vi "Main.vi"() -> ()   [LabVIEW 2015]
doc: "This template is for the Queued Message Handler design pattern.\n\nThe Event Handling Loop generates messages based on user interface actions.\n\nThe Message Handling Loop processes messages generated by the Event Handling Loop, or by other messages. The messages are string values, so new messages can be added easily to the Message Cases case structure in the Message Handling Loop. Each message cluster can also provide an optional value for Message Data, which is a variant that can be converted to whatever message-specific data is required."
uses:
  support/Type Definitions/UI Data.ctl
  support/Message Queue/Message Queue.lvlib
  Support/User Event - EHL Stop/User Event - EHL Stop.lvlib
  support/Message Queue/Enqueue Message (Single).vi
  <vilib>/ErrorRing/Error Ring.xnode
  Model/Model.lvlib
  PLC/PLC.lvlib
  support/Status Logger/Status Log.ctl
  support/Global names.vi
  <vilib>/Utility/error.llb/Error Cluster From Error Code.vi
panel:
  out "Power status":bool
  in  "Abort":bool
  in  "Stop Line":bool
  in  "Start Line":bool
  out "Status":string
  in  "Tab Control":enum32{"Simulation"}(tab)
  in  "Power switch":bool
  in  "Positon":dbl(slide) scale=0.0..20.0
  in  "Dispose":bool
  in  "Pump":bool
  in  "Flow [l/s]":dbl=10.0
  in  "Exit":bool
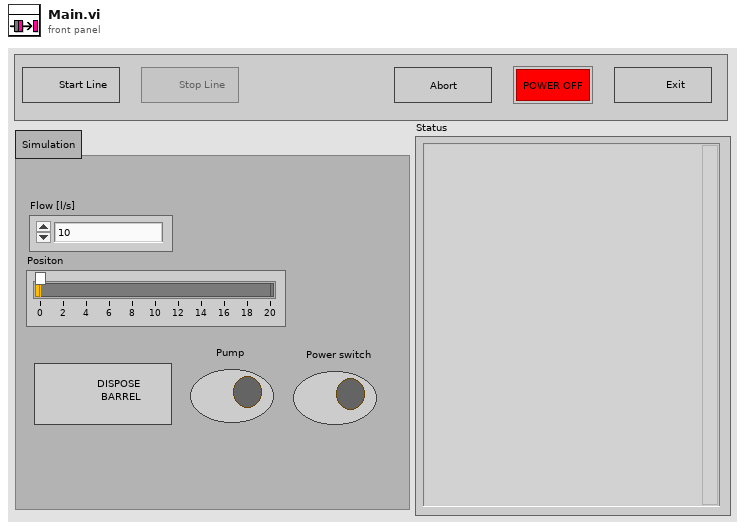
[diagram p1: front panel]
types:
  T1 = typedef "Status Log.ctl" = enum16{"Close file", "Open Status file", "Add Status", "Show Status File"}
  T2 = typedef "UI Data.ctl" = cluster{"Start Line Ref":refnum<vi>, "Stop Line Ref":refnum<vi>, "Data Display Ref":refnum<vi>, "Exit Button Ref":refnum<vi>, "Pump Ref":refnum<vi>, "Dispose Ref":refnum<vi>, "Flow Ref":refnum<vi>, "Position Ref":refnum<vi>, "Tab Ref":refnum<vi>, "Abort":refnum<vi>, "Power status":refnum<vi>, "Power switch":refnum<vi>}
  T3 = typedef "Notifiers.lvlib/Notifiers.ctl" = cluster{"PLC":refnum<notifier>, "Model":refnum<notifier>}
  T4 = typedef "Message Queue.lvlib/All Message Queues.ctl" = cluster{"UI":refnum<queue>, "Model":refnum<queue>, "PLC":refnum<queue>}
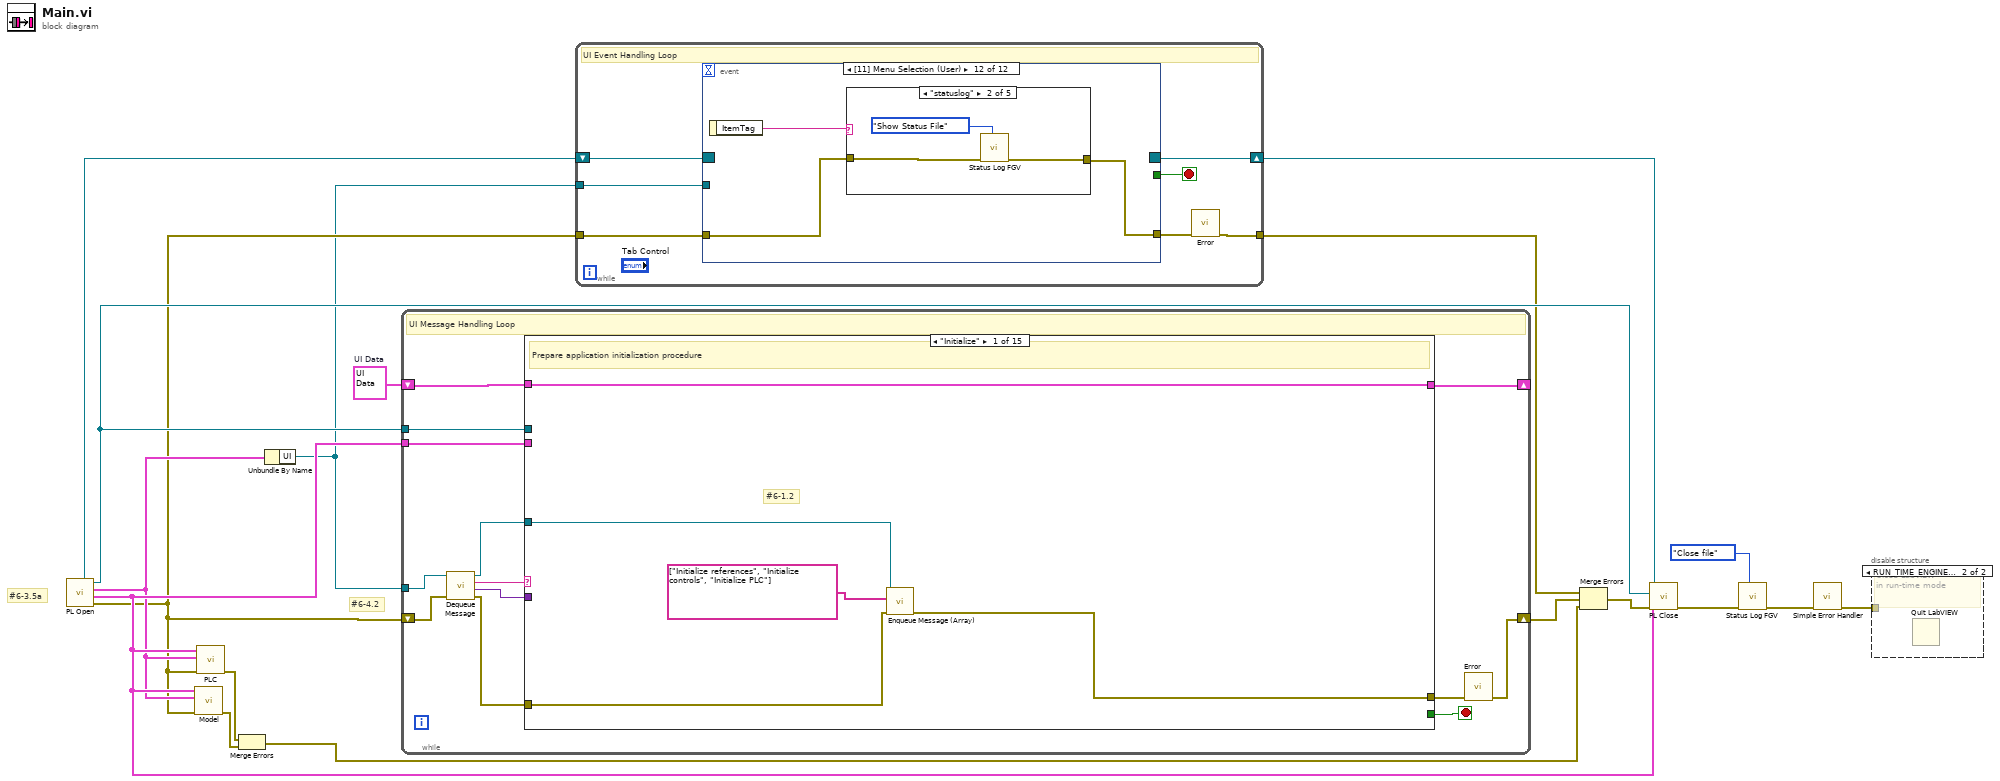
[diagram p0: block diagram]
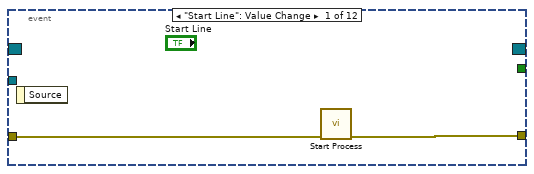
[diagram p2: hidden frame]
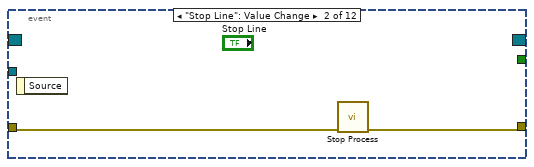
[diagram p3: hidden frame]
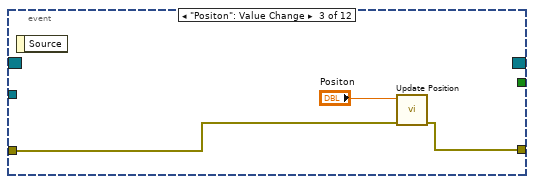
[diagram p4: hidden frame]
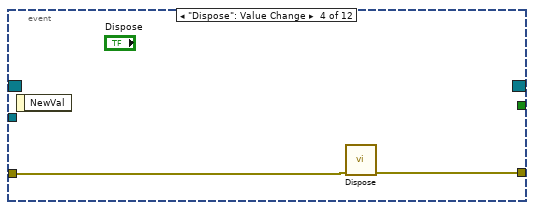
[diagram p5: hidden frame]
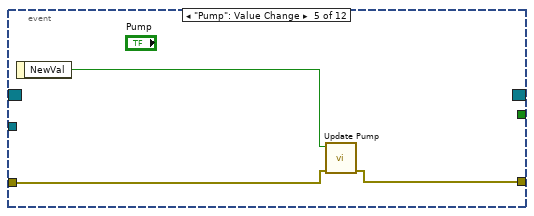
[diagram p6: hidden frame]
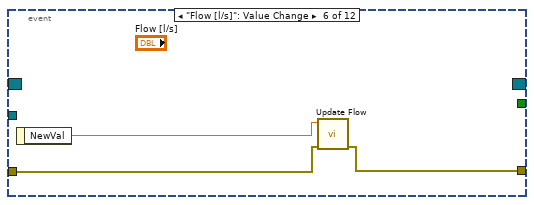
[diagram p7: hidden frame]
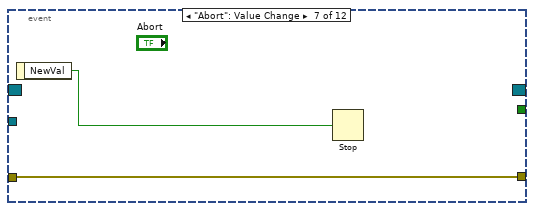
[diagram p8: hidden frame]
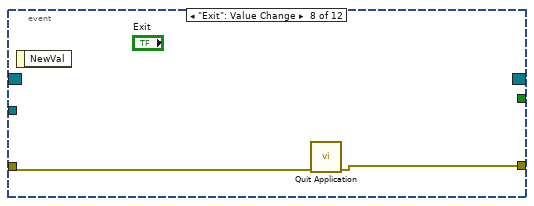
[diagram p9: hidden frame]
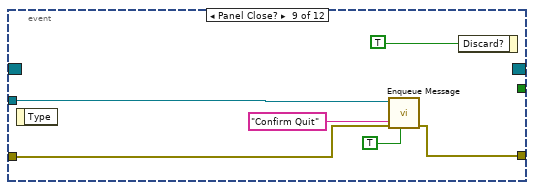
[diagram p10: hidden frame]
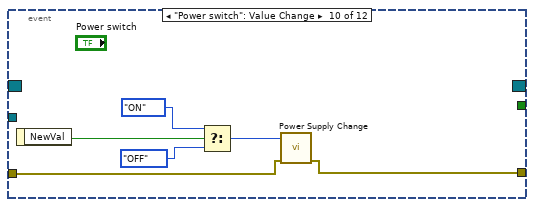
[diagram p11: hidden frame]
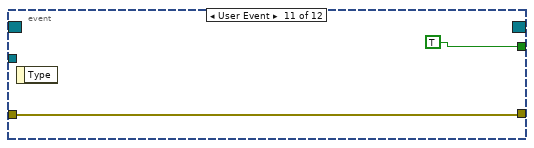
[diagram p12: hidden frame]
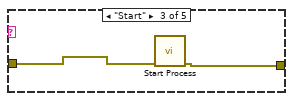
[diagram p14: hidden frame]
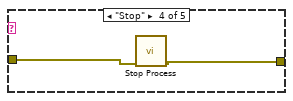
[diagram p15: hidden frame]
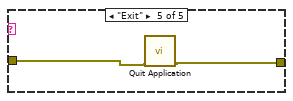
[diagram p16: hidden frame]
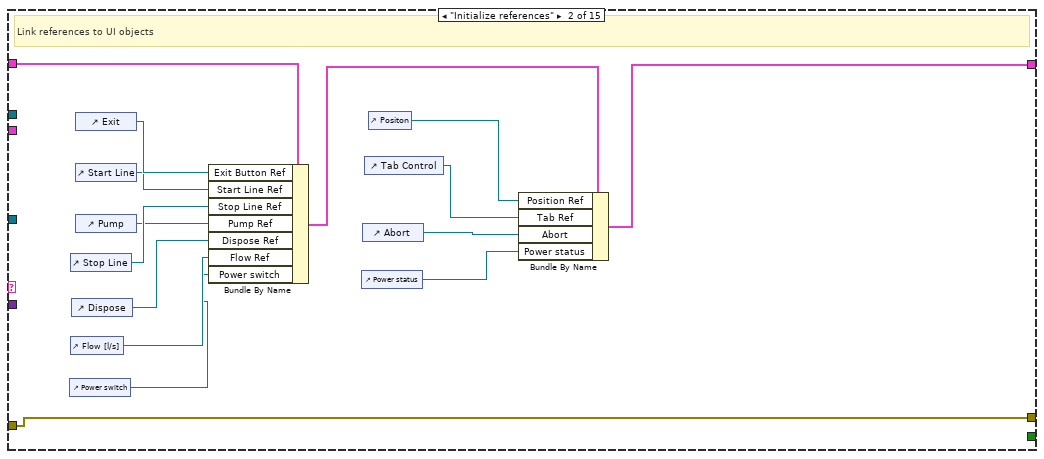
[diagram p18: hidden frame]
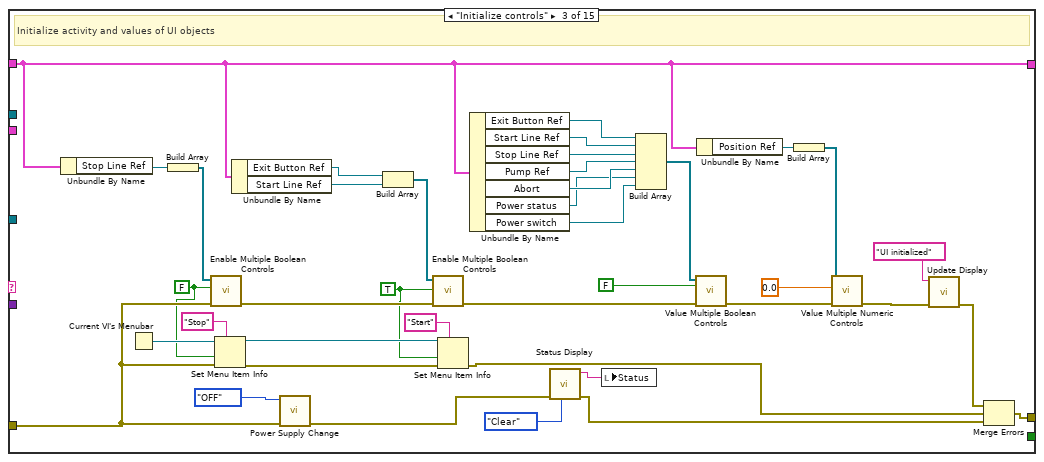
[diagram p19: hidden frame]
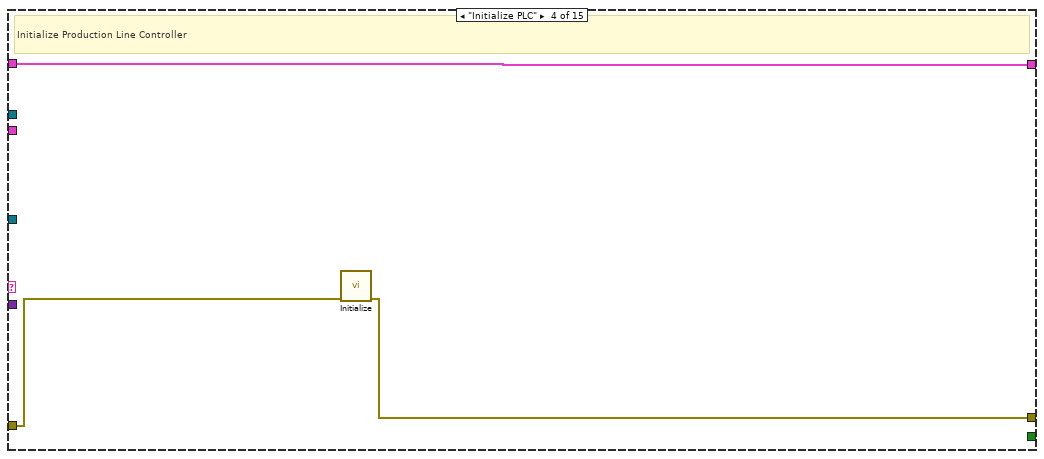
[diagram p20: hidden frame]
diagram:
  w17 = T2 {"Start Line Ref"=refnum, "Stop Line Ref"=refnum, "Data Display Ref"=refnum, "Exit Button Ref"=refnum, "Pump Ref"=refnum, "Dispose Ref"=refnum, "Flow Ref"=refnum, "Position Ref"=refnum, "Tab Ref"=refnum, "Abort"=refnum, "Power status"=refnum, "Power switch"=refnum}  # UI Data
  # "#6-3.5a"
  # "#6-4.2"
  n1 = call "PL Open.vi"() -> ("error out"=w2:errorcluster, "Notifiers"=w7:T3, "Queues"=w6:T4, "User Event"=w15:refnum<user-event>, "Event Registration Refnum"=w9:refnum<event-registration>)  [unwired: 7 in]
  n2 = call "Model.vi"("error in"=w2, "Queues"=w6, "Notifiers"=w7) -> ("error out"=w4:errorcluster)  [unwired: 8 in]
  n3 = call "PLC.vi"("error in"=w2, "Message Queues"=w6, "Notifiers"=w7) -> ("error out"=w5:errorcluster)  [unwired: 8 in]
  n4 = Merge Errors(w5, w4) -> (w3:errorcluster)
  n5 = Unbundle By Name(w6) -> ("UI"=w1:refnum<queue>)
  n6 = while {
    shift-right: [w30] -> _
    shift-left: w17 -> [w31]
    tunnel: w15 -> [w28]
    tunnel: w7 -> [w24]
    shift-right: [w20] -> w13
    shift-left: w2 -> [w27]
    tunnel: w1 -> [w22]
    stop <- w29 stop-if-true
    # "UI Message Handling Loop"
    n7 = call "Dequeue Message.vi"("error in (no error)"=w27, "Message Queue"=w22) -> ("error out"=w26:errorcluster, "Message Data"=w23:variant, "Message"=w19:string, "dup Message Queue"=w25:refnum<queue>)  [unwired: 6 in]
    n8 = case "Message Cases" shown="\"Initialize\"" w19 {
      selector: w19 -> [_ _ _ _ _ _ _ _ _ _ _ _ _ _ w245]
      tunnel: w25 -> [w34 _ _ _ _ _ _ _ _ _ w191 w197 w233 _ _]
      tunnel: w26 -> [w35 w40 w60 w91 w107 w125 w138 w153 w181 w183 w192 w199 w216 w240 _]
      tunnel: [w33 w40 w69 w92 w106 w127 w140 w154 w175 w182 w189 w196 w220 w234 w244] -> w21
      tunnel: w31 -> [w36 w51 w77 w93 w112 w137 w145 w157 w178 w187 w193 w203 w225 w239 w246]
      tunnel: [w36 w41 w77 w93 w112 w137 w145 w157 w178 w187 w193 w203 w225 w239 w246] -> w30
      tunnel: [_ _ _ _ _ _ _ _ _ _ _ _ TRUE _ _] -> w29
      tunnel: w23 -> [_ _ _ _ _ _ w148 w151 w180 w186 _ _ w227 _ _]
      tunnel: w28 -> [_ _ _ _ _ _ _ _ _ _ _ _ w230 _ _]
      tunnel: w24 -> [_ _ _ _ _ _ _ _ _ _ _ w202 _ _ _]
      frame "Initialize" {
        # "#6-1.2"
        # "Prepare application initialization procedure"
        n9 = call "Enqueue Message (Array).vi"("error in (no error)"=w35, "Message Array"=string[] ["Initialize references", "Initialize controls", "Initialize PLC"], "Message Queue"=w34) -> ("error out"=w33:errorcluster)  [unwired: 7 in, 1 out]
      }
      frame "Initialize references" {
        # "Link references to UI objects"
        n10 = control-ref of="Power switch"() -> (w39:refnum<vi>)
        n11 = control-ref of="Stop Line"() -> (w48:refnum<vi>)
        n12 = control-ref of="Flow [l/s]"() -> (w45:refnum<vi>)
        n13 = control-ref of="Dispose"() -> (w46:refnum<vi>)
        n14 = control-ref of="Exit"() -> (w50:refnum<vi>)
        n15 = control-ref of="Start Line"() -> (w49:refnum<vi>)
        n16 = control-ref of="Pump"() -> (w47:refnum<vi>)
        n17 = Bundle By Name(cluster=w51, "Exit Button Ref"=w50, "Start Line Ref"=w49, "Stop Line Ref"=w48, "Pump Ref"=w47, "Dispose Ref"=w46, "Flow Ref"=w45, "Power switch"=w39) -> (w44:T2)
        n18 = control-ref of="Power status"() -> (w37:refnum<vi>)
        n19 = control-ref of="Abort"() -> (w38:refnum<vi>)
        n20 = control-ref of="Tab Control"() -> (w42:refnum<vi>)
        n21 = control-ref of="Positon"() -> (w43:refnum<vi>)
        n22 = Bundle By Name(cluster=w44, "Position Ref"=w43, "Tab Ref"=w42, "Abort"=w38, "Power status"=w37) -> (w41:T2)
      }
      frame "Initialize controls" {
        w52 = TRUE ("Enabled")
        w53 = FALSE ("Enabled")
        # "Initialize activity and values of UI objects"
        n23 = Unbundle By Name(w77) -> ("Stop Line Ref"=w90:refnum<vi>)
        n24 = Current VI's Menubar() -> (w55:refnum<k9>)
        n25 = Build Array(w90) -> (w89:refnum<vi>[])
        n26 = call "Enable Multiple Boolean Controls.vi"("error in"=w60, "Enabled"=w53, "References"=w89) -> ("error out"=w86:errorcluster)  [unwired: 8 in]
        n27 = Set Menu Item Info(7:"Stop" ("item tag"), 8:w60, 9:w53, 11:w55) -> (0:w58:errorcluster, 3:w54:refnum<k9>)  [unwired: 3 in]
        n28 = Unbundle By Name(w77) -> ("Exit Button Ref"=w88:refnum<vi>, "Start Line Ref"=w87:refnum<vi>)
        n29 = call "Power Supply Change.vi"("error in"=w60, "Power status"=enum16{"OFF", "ON"}."OFF") -> ("error out"=w66:errorcluster)  [unwired: 9 in]
        n30 = Build Array(w88, w87) -> (w85:refnum<vi>[])
        n31 = call "Enable Multiple Boolean Controls.vi"("error in"=w86, "Enabled"=w52, "References"=w85) -> ("error out"=w80:errorcluster)  [unwired: 8 in]
        n32 = Set Menu Item Info(7:"Start" ("item tag"), 8:w58, 9:w52, 11:w54) -> (0:w56:errorcluster)  [unwired: 3 in, 1 out]
        n33 = Unbundle By Name(w77) -> ("Exit Button Ref"=w84:refnum<vi>, "Start Line Ref"=w83:refnum<vi>, "Stop Line Ref"=w82:refnum<vi>, "Pump Ref"=w81:refnum<vi>, "Abort"=w72:refnum<vi>, "Power status"=w71:refnum<vi>, "Power switch"=w62:refnum<vi>)
        n34 = call "Status Display.vi"("Action"=enum16{"Update", "Clear"}."Clear", "error in"=w66) -> ("error out"=w65:errorcluster, "Status"=w63:string)  [unwired: 8 in]
        n35 = local write "Status"(w63) -> ()
        n36 = Build Array(w84, w83, w82, w81, w72, w71, w62) -> (w78:refnum<vi>[])
        n37 = call "Value Multiple Boolean Controls.vi"("error in"=w80, "Value"=FALSE ("Enabled"), "References"=w78) -> ("error out"=w76:errorcluster)  [unwired: 8 in]
        n38 = Unbundle By Name(w77) -> ("Position Ref"=w75:refnum<vi>)
        n39 = Build Array(w75) -> (w74:refnum<vi>[])
        n40 = call "Value Multiple Numeric Controls.vi"("error in"=w76, "Value"=0.0, "References"=w74) -> ("error out"=w68:errorcluster)  [unwired: 8 in]
        n41 = call "Update Display.vi"("error in"=w68, "Message string"="UI initialized") -> ("error out"=w57:errorcluster)  [unwired: 9 in]
        n42 = Merge Errors(w57, w56, w65) -> (w69:errorcluster)
      }
      frame "Initialize PLC" {
        # "Initialize Production Line Controller"
        n43 = call "Initialize.vi"("error in"=w91) -> ("error out"=w92:errorcluster)  [unwired: 10 in]
      }
      frame "Start process" {
        w98 = TRUE ("Enabled")
        w102 = FALSE ("Enabled")
        # "Starts process: start PLC, open logger file, create reports files, enable/disable UI controls and update status display"
        n44 = Unbundle By Name(w112) -> ("Exit Button Ref"=w95:refnum<vi>, "Start Line Ref"=w108:refnum<vi>, "Stop Line Ref"=w111:refnum<vi>)
        n45 = Build Array(w95, w108) -> (w113:refnum<vi>[])
        n46 = Build Array(w111) -> (w110:refnum<vi>[])
        n47 = call "Start.vi"("error in"=w107) -> ("error out"=w109:errorcluster)  [unwired: 10 in]
        n48 = call "Enable Multiple Boolean Controls.vi"("error in"=w107, "Enabled"=w98, "References"=w110) -> ("error out"=w100:errorcluster)  [unwired: 8 in]
        n49 = call "Enable Multiple Boolean Controls.vi"("error in"=w107, "Enabled"=w102, "References"=w113) -> ("error out"=w104:errorcluster)  [unwired: 8 in]
        n50 = global read "Global names.vi" "Starting"() -> (w96:string)
        n51 = Current VI's Menubar() -> (w97:refnum<k9>)
        n52 = call "Update Display.vi"("error in"=w109, "Message string"=w96) -> ("error out"=w94:errorcluster)  [unwired: 9 in]
        n53 = Set Menu Item Info(7:"Start" ("item tag"), 8:w104, 9:w102, 11:w97) -> (0:w103:errorcluster)  [unwired: 3 in, 1 out]
        n54 = Set Menu Item Info(7:"Stop" ("item tag"), 8:w100, 9:w98, 11:w97) -> (0:w99:errorcluster)  [unwired: 3 in, 1 out]
        n55 = Merge Errors(w94, w103, w99) -> (w106:errorcluster)
      }
      frame "Stop process" {
        w116 = FALSE ("Enabled")
        w117 = TRUE ("Enabled")
        # "Stops process: stop PLC, close logger file, save and close report files, enable/disable UI controls and update status display"
        n56 = Unbundle By Name(w137) -> ("Exit Button Ref"=w114:refnum<vi>, "Start Line Ref"=w130:refnum<vi>, "Stop Line Ref"=w136:refnum<vi>)
        n57 = call "Stop.vi"("error in"=w125) -> ("error out"=w132:errorcluster)  [unwired: 10 in]
        n58 = Build Array(w136) -> (w126:refnum<vi>[])
        n59 = Build Array(w114, w130) -> (w134:refnum<vi>[])
        n60 = global read "Global names.vi" "Stopping"() -> (w115:string)
        n61 = Build Array (concatenate)(w134, w126) -> (w133:refnum<vi>[])
        n62 = call "Enable Multiple Boolean Controls.vi"("error in"=w125, "Enabled"=w117, "References"=w134) -> ("error out"=w122:errorcluster)  [unwired: 8 in]
        n63 = call "Enable Multiple Boolean Controls.vi"("error in"=w125, "Enabled"=w116, "References"=w126) -> ("error out"=w129:errorcluster)  [unwired: 8 in]
        n64 = call "Value Multiple Boolean Controls.vi"("error in"=w125, "Value"=FALSE, "References"=w133) -> ("error out"=w128:errorcluster)  [unwired: 8 in]
        n65 = call "Update Display.vi"("error in"=w132, "Message string"=w115) -> ("error out"=w131:errorcluster)  [unwired: 9 in]
        n66 = Current VI's Menubar() -> (w123:refnum<k9>)
        n67 = Set Menu Item Info(7:"Start" ("item tag"), 8:w122, 9:w117, 11:w123) -> (0:w120:errorcluster, 3:w118:refnum<k9>)  [unwired: 3 in]
        n68 = Set Menu Item Info(7:"Stop" ("item tag"), 8:w120, 9:w116, 11:w118) -> (0:w119:errorcluster)  [unwired: 3 in, 1 out]
        n69 = Merge Errors(w131, w119, w129, w128) -> (w127:errorcluster)
      }
      frame "Update display" {
        # "#6-3.5b"
        # "Updates status display, status log file and word report file"
        n70 = Variant To Data(error in=w138, type="", Variant=w148) -> (data=w139:string, error out=w142:errorcluster)
        n71 = call "Status Display.vi"("Action"=enum16{"Update", "Clear"}."Update", "error in"=w142, "Status line"=w139) -> ("error out"=w141:errorcluster, "Status"=→"Status":string)  [unwired: 7 in]
        n72 = property on="Status" class="Str"("Text.Scroll Position"=-1) -> ()  [unwired: 2 in, 2 out]
        n73 = Merge Errors(w138, w141) -> (w140:errorcluster)
      }
      frame "Update position" {
        # "Programmatically update position of the barrel slider"
        n74 = Variant To Data(error in=w153, type=0.0 ("Value"), Variant=w151) -> (data=w149:dbl, error out=w152:errorcluster)
        n75 = Unbundle By Name(w157) -> ("Position Ref"=w156:refnum<vi>)
        n76 = Build Array(w156) -> (w155:refnum<vi>[])
        n77 = call "Value Multiple Numeric Controls.vi"("error in"=w152, "Value"=w149, "References"=w155) -> ("error out"=w154:errorcluster)  [unwired: 8 in]
      }
      frame "Power status change" {
        # "Update main switch LED and Start/Stop buttons according to power status change (DAQ DI)"
        n78 = Variant To Data(error in=w181, type=TRUE, Variant=w180) -> (data=w158:bool, error out=w162:errorcluster)
        "Power status" <- w158
        n79 = Unbundle By Name(w178) -> ("Start Line Ref"=w177:refnum<vi>, "Stop Line Ref"=w176:refnum<vi>)
        n80 = Build Array(w177) -> (w174:refnum<vi>[])
        n81 = Build Array(w176) -> (w171:refnum<vi>[])
        n82 = Build Array (concatenate)(w174, w171) -> (w173:refnum<vi>[])
        n83 = Current VI's Menubar() -> (w165:refnum<k9>)
        n84 = call "Enable Multiple Boolean Controls.vi"("error in"=w162, "Enabled"=w158, "References"=w174) -> ("error out"=w169:errorcluster)  [unwired: 8 in]
        n85 = Set Menu Item Info(7:"Start" ("item tag"), 8:w162, 9:w158, 11:w165) -> (0:w163:errorcluster, 3:w159:refnum<k9>)  [unwired: 3 in]
        n86 = call "Value Multiple Boolean Controls.vi"("error in"=w162, "Value"=FALSE, "References"=w173) -> ("error out"=w168:errorcluster)  [unwired: 8 in]
        n87 = call "Enable Multiple Boolean Controls.vi"("error in"=w162, "Enabled"=FALSE, "References"=w171) -> ("error out"=w167:errorcluster)  [unwired: 8 in]
        n88 = Set Menu Item Info(7:"Stop" ("item tag"), 8:w163, 9:FALSE ("enabled"), 11:w159) -> (0:w160:errorcluster)  [unwired: 3 in, 1 out]
        n89 = Merge Errors(w169, w168, w167, w160) -> (w175:errorcluster)
      }
      frame "Error" {
        # "Display error dialog box and quit application"
        n90 = Variant To Data(error in=w183, type=errorcluster {"status"=FALSE, "code"=0, "source"=""} ("error constant"), Variant=w186) -> (data=w184:errorcluster, error out=w182:errorcluster)
        n91 = call <vilib>:"Simple Error Handler.vi"("error in (no error)"=w184) -> ()  [unwired: 4 in, 5 out]
      }
      frame "Exit" {
        # "Start exit procedure: stop PLC, then send Exit message to PLC and go to PLC confirmation loop"
        n92 = Flush Queue(queue=w191, error in (no error)=w192) -> (error out=w188:errorcluster)  [unwired: 2 out]
        n93 = call "Exit PLC.vi"("error in"=w188) -> ("error out"=w190:errorcluster)  [unwired: 10 in]
        n94 = call "Wait on PLC Exit.vi"("error in"=w190) -> ("error out"=w189:errorcluster)  [unwired: 10 in]
      }
      frame "Wait on PLC exit" {
        # "Wait until PLC shutdown"
        n95 = Unbundle By Name(w202) -> ("PLC"=w201:refnum<notifier>)
        n96 = Wait on Notification(notifier=w201, timeout in ms (-1)=10, error in (no error)=w199) -> (notification=w195:string, timed out?=w198:bool, error out=w194:errorcluster)  [unwired: 1 in, 1 out]
        n97 = case shown="True" w198 {
          tunnel: [w204 w213] -> w196
          tunnel: w194 -> [w205 w210]
          tunnel: w197 -> [_ w211]
          tunnel: w195 -> [_ w206]
          frame True {
            # "Shutdown notification from PLC not received"
            n98 = call "Wait on PLC Exit.vi"("error in"=w205) -> ("error out"=w204:errorcluster)  [unwired: 10 in]
          }
          frame False {
            # "Shutdown notification from PLC received (handshake)"
            n99 = call "Update Display.vi"("error in"=w210, "Message string"=w206) -> ("error out"=w209:errorcluster)  [unwired: 9 in]
            n100 = call "Update Display.vi"("error in"=w209, "Message string"="Application quits" ("Message")) -> ("error out"=w208:errorcluster)  [unwired: 9 in]
            n101 = call-poly "Enqueue Message.vi"("error in (no error)"=w208, "Message"="End program", "Message Queue"=w211) -> ("error out"=w213:errorcluster)  [unwired: 7 in, 1 out]
          }
        }
      }
      frame "End program" {
        # "Shutdown MHL and send exit user event to EHL; reset UI controls"
        n102 = call "Fire User Event - EHL Stop.vi"("error in (no error)"=w216, "User Event - Stop"=w230) -> ("error out"=w215:errorcluster)  [unwired: 9 in]
        n103 = Variant To Data(error in=w216, type=errorcluster {"status"=FALSE, "code"=0, "source"=""} ("error constant"), Variant=w227) -> (data=w228:errorcluster)  [unwired: 1 out]
        n104 = Release Queue(queue=w233, force destroy? (F)=TRUE, error in (no error)=w216) -> (error out=w231:errorcluster)  [unwired: 2 out]
        n105 = call <vilib>:"Simple Error Handler.vi"("error in (no error)"=w228) -> ("error out"=w214:errorcluster)  [unwired: 4 in, 4 out]
        n106 = Merge Errors(w215, w214, w231) -> (w221:errorcluster)
        n107 = Unbundle By Name(w225) -> ("Exit Button Ref"=w224:refnum<vi>, "Abort"=w219:refnum<vi>, "Start Line Ref"=w218:refnum<vi>, "Stop Line Ref"=w217:refnum<vi>)
        n108 = Build Array(w224, w219, w218, w217) -> (w223:refnum<vi>[])
        n109 = call "Value Multiple Boolean Controls.vi"("error in"=w221, "Value"=FALSE, "References"=w223) -> ("error out"=w220:errorcluster)  [unwired: 8 in]
      }
      frame "Confirm Quit" {
        # "Confirm Quit - Message that can confirm whether or not the user wants to exit the application."
        n110 = Two Button Dialog(message="Are you sure?", 1:"Continue" ("F button name (\"Cancel\")"), 2:"Quit" ("T button name (\"OK\")")) -> (T button?=w235:bool)
        n111 = case shown="True" w235 {
          tunnel: w240 -> [w241 w243]
          tunnel: [w241 w242] -> w234
          frame False {
          }
          frame True {
            n112 = call "Quit Application.vi"("error in"=w243) -> ("error out"=w242:errorcluster)  [unwired: 10 in]
          }
        }
      }
      frame Default {
        # "Incorrect message: show error and clear error"
        n113 = xnode "Error Ring"("parameter 0"=w245) -> ("error out"=w244:errorcluster)
      }
    }
    n114 = call "Error.vi"("error in"=w21) -> ("error out"=w20:errorcluster)  [unwired: 10 in]
  }
  n115 = while {
    tunnel: w1 -> [w256]
    shift-right: [w259] -> w18
    shift-left: w9 -> [w260]
    tunnel: [w254] -> w8
    tunnel: w2 -> [w257]
    stop <- w258 stop-if-true
    # "UI Event Handling Loop"
    n116 = event shown="[11] Menu Selection (User)" {
      selector: w260 -> [_ _ _ _ _ _ _ _ _ _ _ _]
      dyn-events: [_ _ _ _ _ _ _ _ _ _ _ _] -> w259
      timeout: _ -> [_ _ _ _ _ _ _ _ _ _ _ _]
      tunnel: [_ _ _ _ _ _ _ _ _ _ TRUE ("Discard?") _] -> w258
      tunnel: w256 -> [_ _ _ _ _ _ _ _ w285 _ _ _]
      tunnel: [w261 w263 w266 w268 w271 w274 w277 w278 w284 w286 w292 w295] -> w255
      tunnel: w257 -> [w262 w264 w265 w269 w272 w275 w277 w279 w280 w287 w292 w294]
      event "Start Line": Value Change {
        n117 = event-data() -> ()  [unwired: 1 in, 1 out]
        n118 = call "Start Process.vi"("error in"=w262) -> ("error out"=w261:errorcluster)  [unwired: 10 in]
      }
      event "Stop Line": Value Change {
        n119 = event-data() -> ()  [unwired: 1 in, 1 out]
        n120 = call "Stop Process.vi"("error in"=w264) -> ("error out"=w263:errorcluster)  [unwired: 10 in]
      }
      event "Positon": Value Change {
        n121 = event-data() -> ()  [unwired: 1 in, 1 out]
        n122 = call "Update Position.vi"("error in (no error)"=w265, "Position"="Positon") -> ("error out"=w266:errorcluster)  [unwired: 9 in]
      }
      event "Dispose": Value Change {
        n123 = event-data() -> ()  [unwired: 1 in, 1 out]
        n124 = call "Dispose.vi"("error in (no error)"=w269) -> ("error out"=w268:errorcluster)  [unwired: 10 in]
      }
      event "Pump": Value Change {
        n125 = event-data() -> ("NewVal"=w270:bool)  [unwired: 1 in]
        n126 = call "Update Pump.vi"("error in (no error)"=w272, "Pump State"=w270) -> ("error out"=w271:errorcluster)  [unwired: 9 in]
      }
      event "Flow [l/s]": Value Change {
        n127 = event-data() -> ("NewVal"=w273:dbl)  [unwired: 1 in]
        n128 = call "Update Flow.vi"("error in (no error)"=w275, "Flow"=w273) -> ("error out"=w274:errorcluster)  [unwired: 9 in]
      }
      event "Abort": Value Change {
        n129 = event-data() -> ("NewVal"=w276:bool)  [unwired: 1 in]
        n130 = Stop(stop? (T)=w276) -> ()
      }
      event "Exit": Value Change {
        n131 = event-data() -> ()  [unwired: 1 in, 1 out]
        n132 = call "Quit Application.vi"("error in"=w279) -> ("error out"=w278:errorcluster)  [unwired: 10 in]
      }
      event Panel Close? {
        n133 = event-data() -> ()  [unwired: 1 in, 1 out]
        n134 = call-poly "Enqueue Message.vi"("Priority Message? (F)"=TRUE, "error in (no error)"=w280, "Message"="Confirm Quit", "Message Queue"=w285) -> ("error out"=w284:errorcluster)  [unwired: 6 in, 1 out]
        n135 = event-data("Discard?"=TRUE) -> ()  [unwired: 1 in, 1 out]
      }
      event "Power switch": Value Change {
        n136 = event-data() -> ("NewVal"=w291:bool)  [unwired: 1 in]
        n137 = Select(t=enum16{"OFF", "ON"}."ON" ("Power status"), s=w291, f=enum16{"OFF", "ON"}."OFF" ("Power status")) -> (s? t:f=w288:enum16{"OFF", "ON"})
        n138 = call "Power Supply Change.vi"("error in"=w287, "Power status"=w288) -> ("error out"=w286:errorcluster)  [unwired: 9 in]
      }
      event User Event {
        n139 = event-data() -> ()  [unwired: 1 in, 1 out]
      }
      event Menu Selection (User) {
        n140 = event-data() -> ("ItemTag"=w296:string)  [unwired: 1 in]
        n141 = case shown="\"statuslog\"" w296 {
          tunnel: [w297 w298 w302 w303 w305] -> w295
          tunnel: w294 -> [w297 w299 w301 w304 w306]
          frame Default {
          }
          frame "statuslog" {
            n142 = call "Status Log FGV.vi"("Action"=Status_Log."Show Status File", "error in"=w299) -> ("error out"=w298:errorcluster)  [unwired: 9 in]
          }
          frame "Start" {
            n143 = call "Start Process.vi"("error in"=w301) -> ("error out"=w302:errorcluster)  [unwired: 10 in]
          }
          frame "Stop" {
            n144 = call "Stop Process.vi"("error in"=w304) -> ("error out"=w303:errorcluster)  [unwired: 10 in]
          }
          frame "Exit" {
            n145 = call "Quit Application.vi"("error in"=w306) -> ("error out"=w305:errorcluster)  [unwired: 10 in]
          }
        }
      }
    }
    n146 = call "Error.vi"("error in"=w255) -> ("error out"=w254:errorcluster)  [unwired: 10 in]
  }
  n147 = Merge Errors(w8, w13, w3) -> (w12:errorcluster)
  n148 = call "PL Close.vi"("error in"=w12, "Notifiers"=w7, "User Event"=w15, "Event Registration Refnum in"=w18) -> ("error out"=w16:errorcluster)  [unwired: 7 in]
  n149 = call "Status Log FGV.vi"("Action"=Status_Log."Close file", "error in"=w16) -> ("error out"=w10:errorcluster)  [unwired: 9 in]
  n150 = call <vilib>:"Simple Error Handler.vi"("error in (no error)"=w10) -> ("error out"=w11:errorcluster)  [unwired: 4 in, 4 out]
  n151 = disable-structure shown="RUN_TIME_ENGINE==True" {
    disable-tunnel: w11 -> [_ _]
    frame condition #0 (active) {
    }
    frame condition #1 {
      # "Close LabVIEW\nin run-time mode"
      n152 = Quit LabVIEW() -> ()  [unwired: 1 in]
    }
  }
